vi "PH_AxisGUI_6P.InitFrontPanel.vi"(0 "i ref in":refnum<vi>, 2 "AxisSelection":refnum<vi>, 5 "error in":errorcluster) -> (14 "i ref out":refnum<vi>, 19 "error out":errorcluster)   [LabVIEW 2014, in "PH_AxisGUI_6P.lvlib"]
doc: "This VI manipulates several GUI elements"
uses:
  PH_AxisGUI_6P.lvlib
  PH_Basics/PH_AxisGUI_BaseClass/PH_AxisGUI_BaseClass.lvlib
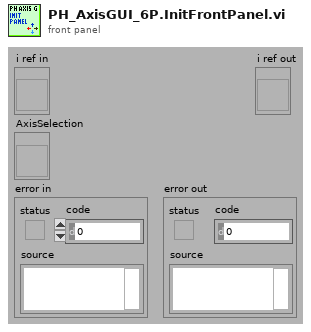
[diagram p1: front panel]
types:
  T1 = typedef "PH_AxisGUI_BaseClass.lvlib/PH_AxisGUI_BaseClass.i attribute.ctl" = cluster{"Axes":T2[]}
  T2 = typedef "PH_AxisGUI_BaseClass.lvlib/PH_AxisGUI_BaseClass.Axis Attributes.ctl" = cluster{"Axis GUI Refs":T3, "Address":T4, "Name":string, "Label \"Back\"":string, "Labell \"Forth\"":string, "Moving?":bool}
  T3 = typedef "PH_AxisGUI_BaseClass.lvlib/PH_AxisGUI_BaseClass.Axis GUI Refs.ctl" = cluster{"Back":refnum<vi>, "Forth":refnum<vi>, "Status":refnum<vi>, "Target":refnum<vi>, "Address":refnum<vi>, "Status Bar":refnum<vi>, "Settings":refnum<vi>, "Activity":refnum<vi>, "Clear Error":refnum<vi>}
  T4 = typedef "PH_Stepmotor_BaseClass.lvlib/PH_Stepmotor_BaseClass.Axis Address.ctl" = cluster{"Instance":string, "Motor Nr":i32}
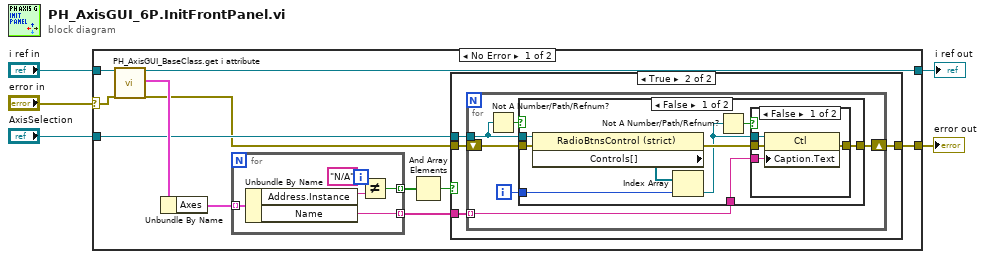
[diagram p0: block diagram]
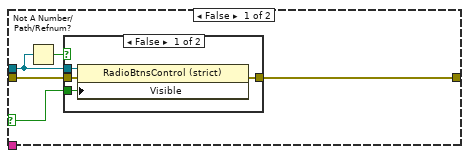
[diagram p2: hidden frame]
diagram:
  n1 = case shown="No Error" "error in" {
    selector: "error in" -> [w13 w57]
    tunnel: "i ref in" -> [w14 w58]
    tunnel: [w16 w58] -> w4
    tunnel: [w15 w57] -> w2
    tunnel: "AxisSelection" -> [w11 _]
    frame No Error {
      n2 = call "PH_AxisGUI_BaseClass.get i attribute.vi"("i ref in"=w14, "error in (no error)"=w13) -> ("i ref out"=w16:refnum<vi>, "i attribute"=w12:T1, "error out"=w10:errorcluster)  [unwired: 15 in]
      n3 = Unbundle By Name(w12) -> ("Axes"=w6:T2[])
      n4 = for {
        tunnel: w6 -> [w54] mode=indexing
        tunnel: [w53] -> w9 mode=indexing
        tunnel: [w52] -> w7 mode=indexing
        n5 = Unbundle By Name(w54) -> ("Address.Instance"=w55:string, "Name"=w52:string)
        n6 = Not Equal?(x="N/A", y=w55) -> (x != y?=w53:bool)
      }
      n7 = And Array Elements(Boolean array=w9) -> (logical AND=w8:bool)
      n8 = case shown="True" w8 {
        selector: w8 -> [w17 _]
        tunnel: [w19 w30] -> w15
        tunnel: w7 -> [_ w29]
        tunnel: w11 -> [w20 w28]
        tunnel: w10 -> [w18 w27]
        frame False {
          n9 = Not A Number/Path/Refnum?(number/path/refnum=w20) -> (NaN/Path/Refnum?=w21:bool)
          n10 = case "Config Axis Selection" shown="False" w21 {
            tunnel: w18 -> [w25 w26]
            tunnel: [w23 w26] -> w19
            tunnel: w20 -> [w24 _]
            tunnel: w17 -> [w22 _]
            frame False {
              n11 = property class="RadioBtnsControl (strict)"(reference=w24, error in=w25, "Visible"=w22) -> (error out=w23:errorcluster)  [unwired: 1 out]
            }
            frame True {
            }
          }
        }
        frame True {
          n12 = for {
            shift-right: [w33] -> w30
            shift-left: w27 -> [w34]
            tunnel: w29 -> [w31] mode=indexing
            tunnel: w28 -> [w32]
            i -> [w35]
            n13 = Not A Number/Path/Refnum?(number/path/refnum=w32) -> (NaN/Path/Refnum?=w36:bool)
            n14 = case "Config Axis Selection" shown="False" w36 {
              tunnel: w34 -> [w39 w51]
              tunnel: w31 -> [w43 _]
              tunnel: [w44 w51] -> w33
              tunnel: w32 -> [w38 _]
              tunnel: w35 -> [w37 _]
              frame False {
                n15 = property class="RadioBtnsControl (strict)"(reference=w38, error in=w39) -> (error out=w45:errorcluster, "Controls[]"=w42:refnum<vi>[])  [unwired: 1 out]
                n16 = Index Array(array=w42, index=w37) -> (element=w41:refnum<vi>)
                n17 = Not A Number/Path/Refnum?(number/path/refnum=w41) -> (NaN/Path/Refnum?=w40:bool)
                n18 = case shown="False" w40 {
                  tunnel: w45 -> [w46 w50]
                  tunnel: [w49 w50] -> w44
                  tunnel: w43 -> [w48 _]
                  tunnel: w41 -> [w47 _]
                  frame False {
                    n19 = property class="Ctl"(reference=w47, error in=w46, "Caption.Text"=w48) -> (error out=w49:errorcluster)  [unwired: 1 out]
                  }
                  frame True {
                  }
                }
              }
              frame True {
              }
            }
          }
        }
      }
    }
    frame Error {
    }
  }
  "error out" <- w2
  "i ref out" <- w4
